vi "Vis Interpolate Points.vi"(7 "Tip out Posit":dbl[](array[numeric])=[0.0, 0.0, 0.0] format="%#.3f") -> (0 "Z":dbl[](array[numeric]) format="%#.3f", 1 "Y":dbl[](array[numeric]) format="%#.3f", 2 "X":dbl[](array[numeric]) format="%#.3f")   [LabVIEW 2016]
uses:
  <vilib>/Analysis/1siggen.llb/Ramp Pattern by Samples.vi
  <vilib>/Analysis/NI_AALBase.lvlib
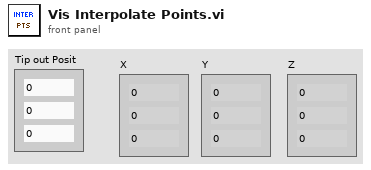
[diagram p1: front panel]
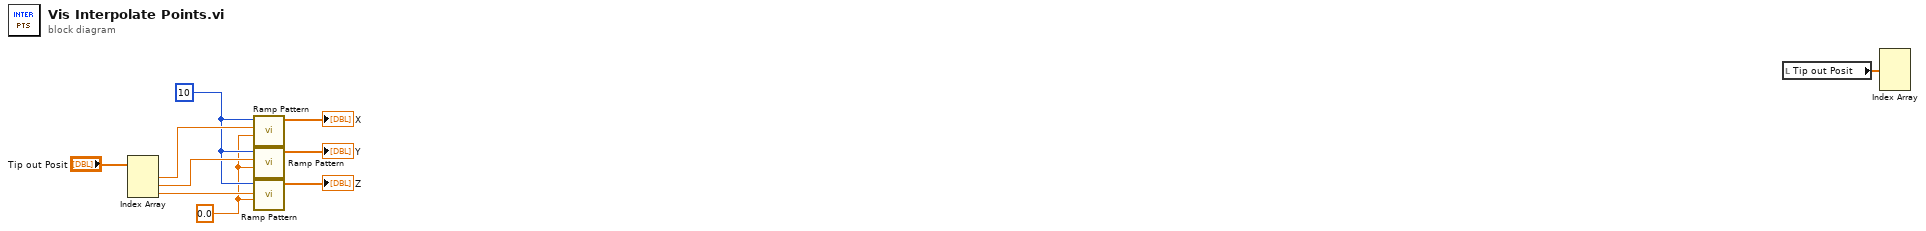
[diagram p0: block diagram]
diagram:
  w4 = 0.0 ("start")
  w5 = 10 ("samples")
  n1 = Index Array(array="Tip out Posit") -> (element #1=w8:dbl, element #2=w7:dbl, element #3=w6:dbl)  [unwired: 3 in]
  n2 = call-poly <vilib>:"Ramp Pattern.vi"("start"=w4, "end"=w8, "samples"=w5) -> ("Ramp Pattern"=→"X":dbl[])  [unwired: 7 in, 1 out]
  n3 = call-poly <vilib>:"Ramp Pattern.vi"("start"=w4, "end"=w7, "samples"=w5) -> ("Ramp Pattern"=→"Y":dbl[])  [unwired: 7 in, 1 out]
  n4 = call-poly <vilib>:"Ramp Pattern.vi"("start"=w4, "end"=w6, "samples"=w5) -> ("Ramp Pattern"=→"Z":dbl[])  [unwired: 7 in, 1 out]
  n5 = local read "Tip out Posit"() -> (w10:dbl[])
  n6 = Index Array(array=w10) -> ()  [unwired: 3 in, 3 out]
